vi "Count Tabs to the Left.vi"(8 "error in":errorcluster, 10 "Current Tab":i32, 11 "Tab Pages References In":refnum<vi>[](array[refnum])) -> (0 "error out":errorcluster, 2 "Number of Tabs to the Left":i32, 3 "Tab Pages References Out":refnum<vi>[](array[refnum]))   [LabVIEW 2017, in "DTacq Plot Display Library.lvlib"]
uses:
  DTacq Plot Display Library.lvlib
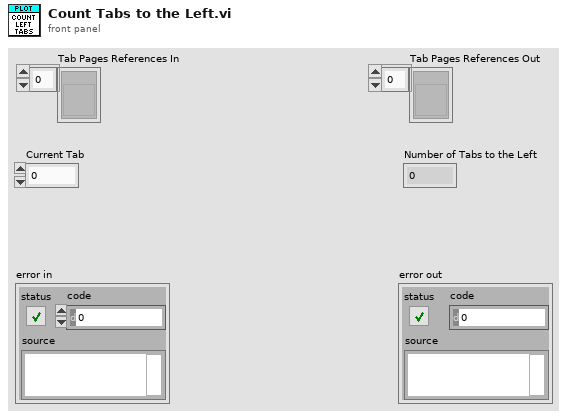
[diagram p1: front panel]
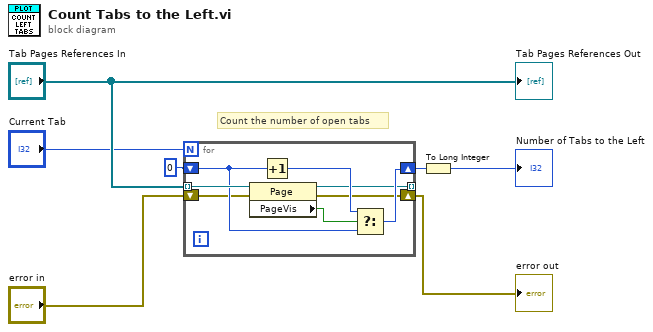
[diagram p0: block diagram]
diagram:
  # "Count the number of open tabs"
  n1 = for {
    N: "Current Tab" -> [_]
    tunnel: "Tab Pages References In" -> [w15] mode=indexing
    shift-right: [w11] -> w6
    shift-left: 0 -> [w12]
    tunnel: [w10] -> _ mode=indexing
    shift-right: [w8] -> w3
    shift-left: "error in" -> [w9]
    n2 = property class="Page"(reference=w15, error in=w9) -> (reference out=w10:refnum<vi>, error out=w8:errorcluster, "PageVis"=w14:bool)
    n3 = Increment(x=w12) -> (x+1=w13:i32)
    n4 = Select(t=w13, s=w14, f=w12) -> (s? t:f=w11:i32)
  }
  "error out" <- w3
  n5 = To Long Integer(number=w6) -> (32bit integer=→"Number of Tabs to the Left":i32)
  "Tab Pages References Out" <- "Tab Pages References In"
